vi "Configure Sweep Time List.vi"(8 "error in (no error)":errorcluster, 10 "Sweep Time List":dbl[](array[numeric])=[0.1, 0.1, 0.1], 11 "VISA resource name":refnum<visa-resource-name>) -> (0 "error out":errorcluster, 3 "VISA resource name out":refnum<visa-resource-name>)   [LabVIEW 2014, in "Agilent MXA Series.lvlib"]
doc: "Cofigures the Sweep Time List under List Sweep measurement type."
uses:
  Agilent MXA Series.lvlib
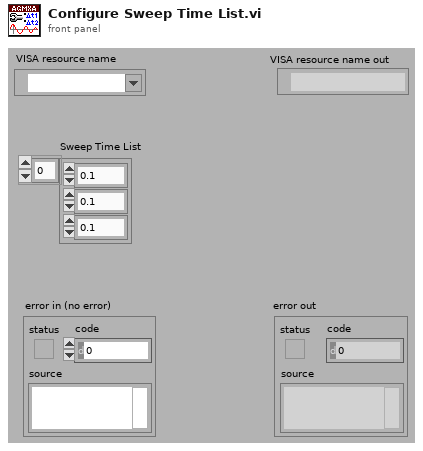
[diagram p1: front panel]
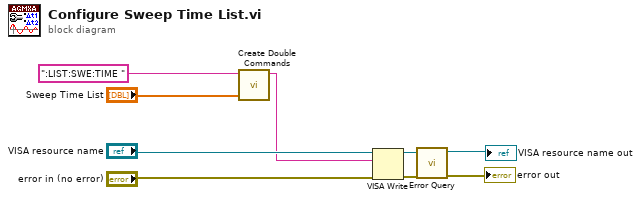
[diagram p0: block diagram]
diagram:
  n1 = call "Create Double Commands.vi"("Double Values"="Sweep Time List", "Commands"=":LIST:SWE:TIME ") -> ("Result"=w1:string)  [unwired: 9 in]
  n2 = VISA Write(VISA resource name="VISA resource name", write buffer=w1, error in (no error)="error in (no error)") -> (VISA resource name out=w8:refnum<visa-resource-name>, error out=w9:errorcluster)  [unwired: 1 out]
  n3 = call "Error Query.vi"("error in (no error)"=w9, "VISA resource name"=w8) -> ("error out"=→"error out":errorcluster, "VISA resource name out"=→"VISA resource name out":refnum<visa-resource-name>)  [unwired: 6 in, 2 out]
